vi "Tank_Monitoring.vi"(8 "Set state:":bool, 10 "Device":T1) -> (0 "Set":bool)   [LabVIEW 2011]
uses:
  Valve_Pump.ctl
  Tank Valves.ctl
  Ordered tank names.ctl
  Pumps_Valves_Dependencies_Global.vi
panel:
  out "Tank Names":string[](array[string])
  out "Happy Tank":bool[](array[boolean])
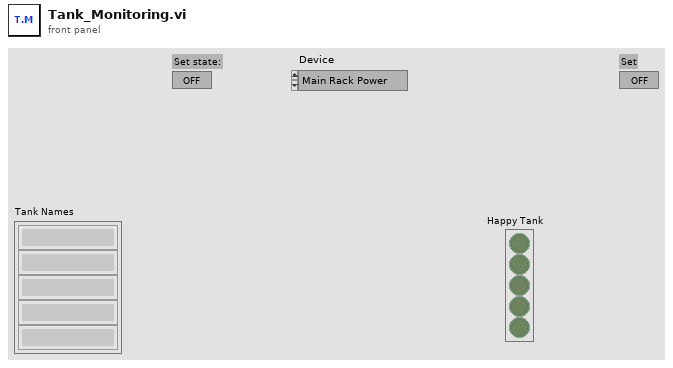
[diagram p1: front panel]
types:
  T1 = typedef "Valve_Pump.ctl" = enum16{"Main Rack Power", "Pump Power", "Valve Power", "V4", "V5", "V6", "V7", "V8", "V9", "V10", "V11", "V12", "V13", "V14", "V15", "V18", "V19", "V20", "V21", "V22", "V23", "V24", "V25", "V26", "V27", "V28", "V29", "V30", "V31", "V32", "V33", "V34", "Pump A", "Pump B", "Pump C", "Pump D"}
  T2 = typedef "Tank Valves.ctl" = enum16{"Salt Saturator", "Tank A", "Tank B", "Tank C", "Tank D"}
  T3 = typedef "Ordered tank names.ctl" = string[]
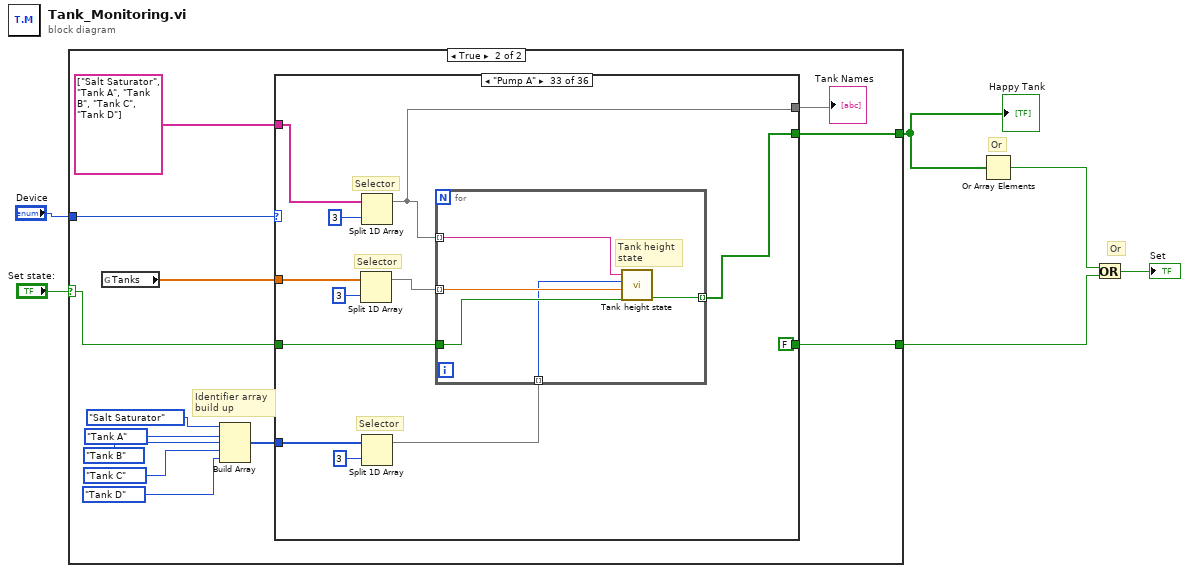
[diagram p0: block diagram]
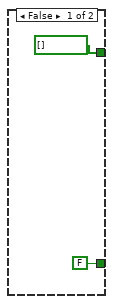
[diagram p2: hidden frame]
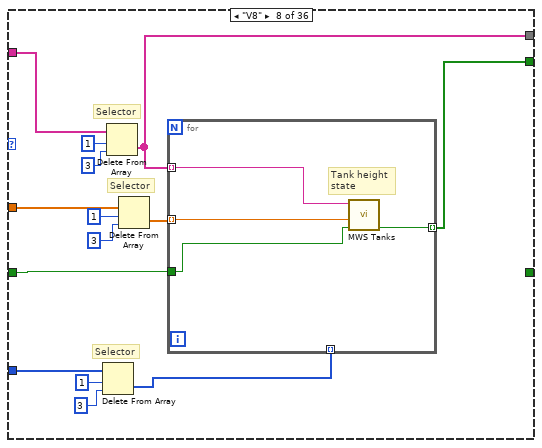
[diagram p10: hidden frame]
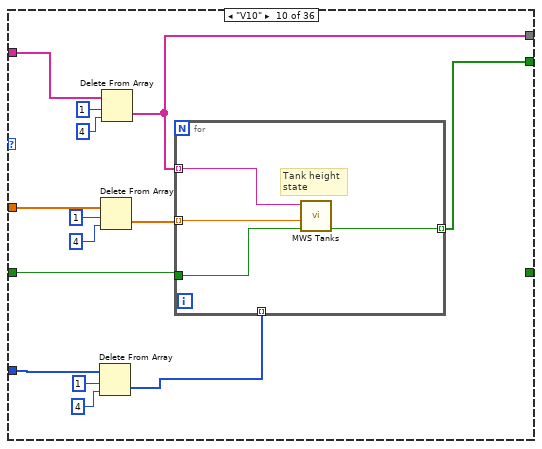
[diagram p12: hidden frame]
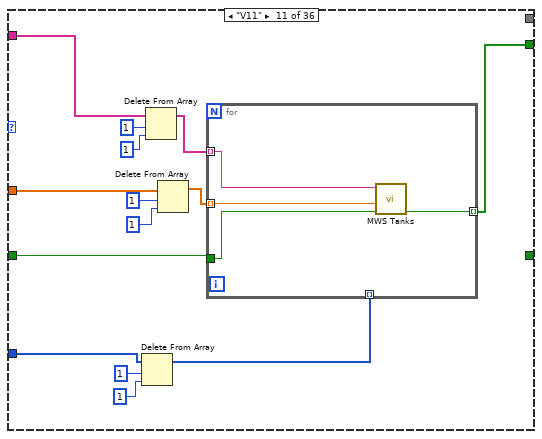
[diagram p13: hidden frame]
diagram:
  # "Or"
  # "Or"
  n1 = case shown="True" "Set state:" {
    selector: "Set state:" -> [_ w11]
    tunnel: [bool[] [] w20] -> w2
    tunnel: [FALSE w10] -> w5
    tunnel: "Device" -> [_ w9]
    frame False {
    }
    frame True {
      # "Identifier array\nbuild up"
      n2 = global read "Pumps_Valves_Dependencies_Global.vi" "Tanks"() -> (w21:dbl[])
      n3 = Build Array(Tank_Valves."Salt Saturator" ("Enum"), Tank_Valves."Tank A" ("Enum"), Tank_Valves."Tank B" ("Enum"), Tank_Valves."Tank C" ("Enum"), Tank_Valves."Tank D" ("Enum")) -> (w12:T2[])
      n4 = case shown="\"Pump A\"" w9 {
        tunnel: w21 -> [_ _ _ _ _ _ _ w35 _ w49 w68 _ _ _ _ _ _ _ _ _ _ _ _ _ _ _ _ _ _ _ _ _ w116 w131 w148 w160]
        tunnel: T3 ["Salt Saturator", "Tank A", "Tank B", "Tank C", "Tank D"] ("Ordered tank names") -> [_ _ _ _ _ _ _ w36 _ w52 w67 _ _ _ _ _ _ _ _ _ _ _ _ _ _ _ _ _ _ _ _ _ w112 w130 w147 w162]
        tunnel: [_ _ _ _ _ _ _ w33 _ w50 w66 _ _ _ _ _ _ _ _ _ _ _ _ _ _ _ _ _ _ _ _ _ w111 w129 w146 w170] -> w20
        tunnel: [_ _ _ _ _ _ _ w31 _ w51 _ _ _ _ _ _ _ _ _ _ _ _ _ _ _ _ _ _ _ _ _ _ w110 w124 w145 w161] -> w18
        tunnel: w12 -> [_ _ _ _ _ _ _ w32 _ w53 w70 _ _ _ _ _ _ _ _ _ _ _ _ _ _ _ _ _ _ _ _ _ w107 w127 w142 w166]
        tunnel: w11 -> [w22 w23 w24 w25 w26 w27 w28 w34 w47 w48 w69 w84 w85 w86 w87 w88 w89 w90 w91 w92 w93 w94 w95 w96 w97 w98 w99 w100 w101 w102 w103 w104 w109 w126 w140 w169]
        tunnel: [w22 w23 w24 w25 w26 w27 w28 _ w47 _ _ w84 w85 w86 w87 w88 w89 w90 w91 w92 w93 w94 w95 w96 w97 w98 w99 w100 w101 w102 w103 w104 FALSE FALSE FALSE FALSE] -> w10
        frame "Main Rack Power" {
        }
        frame "Pump Power" {
        }
        frame "Valve Power" {
        }
        frame "V4" {
        }
        frame "V5" {
        }
        frame "V6" {
        }
        frame "V7" {
        }
        frame "V8" {
          # "Selector"
          # "Selector"
          # "Selector"
          n5 = Delete From Array(array=w32, length=1, index=3) -> (deleted portion=w29:T2[])  [unwired: 1 out]
          n6 = Delete From Array(array=w36, length=1 ("index"), index=3 ("length")) -> (deleted portion=w31:T3)  [unwired: 1 out]
          n7 = Delete From Array(array=w35, length=1 ("index"), index=3 ("length")) -> (deleted portion=w30:dbl[])  [unwired: 1 out]
          n8 = for {
            tunnel: w30 -> [w45] mode=indexing
            tunnel: w31 -> [w44] mode=indexing
            tunnel: [w43] -> w33 mode=indexing
            tunnel: w29 -> [_] mode=indexing
            tunnel: w34 -> [w46]
            # "Tank height\nstate"
            n9 = call "MWS Tanks.vi"("Set state:"=w46, "Tank height"=w45, "Status Message"=w44) -> ("Set"=w43:bool)  [unwired: 8 in]
          }
        }
        frame "V9" {
        }
        frame "V10" {
          n10 = Delete From Array(array=w53, length=1, index=4) -> (deleted portion=w54:T2[])  [unwired: 1 out]
          n11 = Delete From Array(array=w49, length=1 ("index"), index=4 ("length")) -> (deleted portion=w55:dbl[])  [unwired: 1 out]
          n12 = Delete From Array(array=w52, length=1 ("index"), index=4 ("length")) -> (deleted portion=w51:T3)  [unwired: 1 out]
          n13 = for {
            tunnel: w55 -> [w64] mode=indexing
            tunnel: w51 -> [w63] mode=indexing
            tunnel: [w62] -> w50 mode=indexing
            tunnel: w54 -> [_] mode=indexing
            tunnel: w48 -> [w65]
            # "Tank height\nstate"
            n14 = call "MWS Tanks.vi"("Set state:"=w65, "Tank height"=w64, "Status Message"=w63) -> ("Set"=w62:bool)  [unwired: 8 in]
          }
        }
        frame "V11" {
          n15 = Delete From Array(array=w70, length=1, index=1) -> (array with subset deleted=w73:T2[])  [unwired: 1 out]
          n16 = Delete From Array(array=w67, length=1 ("index"), index=1 ("length")) -> (array with subset deleted=w76:T3)  [unwired: 1 out]
          n17 = Delete From Array(array=w68, length=1 ("index"), index=1 ("length")) -> (array with subset deleted=w79:dbl[])  [unwired: 1 out]
          n18 = for {
            tunnel: w79 -> [w82] mode=indexing
            tunnel: w76 -> [w80] mode=indexing
            tunnel: [w83] -> w66 mode=indexing
            tunnel: w73 -> [_] mode=indexing
            tunnel: w69 -> [w81]
            n19 = call "MWS Tanks.vi"("Set state:"=w81, "Tank height"=w82, "Status Message"=w80) -> ("Set"=w83:bool)  [unwired: 8 in]
          }
        }
        frame "V12" {
        }
        frame "V13" {
        }
        frame "V14" {
        }
        frame "V15" {
        }
        frame "V18" {
        }
        frame "V19" {
        }
        frame "V20" {
        }
        frame "V21" {
        }
        frame "V22" {
        }
        frame "V23" {
        }
        frame "V24" {
        }
        frame "V25" {
        }
        frame "V26" {
        }
        frame "V27" {
        }
        frame "V28" {
        }
        frame "V29" {
        }
        frame "V30" {
        }
        frame "V31" {
        }
        frame "V32" {
        }
        frame "V33" {
        }
        frame "V34" {
        }
        frame "Pump A" {
          # "Selector"
          # "Selector"
          # "Selector"
          n20 = Split 1D Array(array=w116, index=3) -> (first subarray=w115:dbl[])  [unwired: 1 out]
          n21 = Split 1D Array(array=w112, index=3) -> (first subarray=w110:T3)  [unwired: 1 out]
          n22 = Split 1D Array(array=w107, index=3) -> (first subarray=w106:T2[])  [unwired: 1 out]
          n23 = for {
            tunnel: w115 -> [w120] mode=indexing
            tunnel: w110 -> [w119] mode=indexing
            tunnel: w109 -> [w121]
            tunnel: [w118] -> w111 mode=indexing
            tunnel: w106 -> [w117] mode=indexing
            # "Tank height\nstate"
            n24 = call "Tank height state.vi"("Set state:"=w121, "Tank height"=w120, "Tank Valves"=w117, "Tank name"=w119) -> ("State"=w118:bool)  [unwired: 6 in]
          }
        }
        frame "Pump B" {
          # "Selector"
          # "Selector"
          # "Selector"
          n25 = Split 1D Array(array=w127, index=1) -> (second subarray=w122:T2[])  [unwired: 1 out]
          n26 = Split 1D Array(array=w131, index=1) -> (second subarray=w123:dbl[])  [unwired: 1 out]
          n27 = Split 1D Array(array=w130, index=1) -> (second subarray=w124:T3)  [unwired: 1 out]
          n28 = for {
            tunnel: w123 -> [w138] mode=indexing
            tunnel: w124 -> [w137] mode=indexing
            tunnel: [w136] -> w129 mode=indexing
            tunnel: w122 -> [w135] mode=indexing
            tunnel: w126 -> [w134]
            # "Tank height\nstate"
            n29 = call "Tank height state.vi"("Set state:"=w134, "Tank height"=w138, "Tank Valves"=w135, "Tank name"=w137) -> ("State"=w136:bool)  [unwired: 6 in]
          }
        }
        frame "Pump C" {
          # "Selector"
          # "Selector"
          # "Selector"
          n30 = Split 1D Array(array=w148, index=3) -> (second subarray=w144:dbl[])  [unwired: 1 out]
          n31 = Split 1D Array(array=w147, index=3) -> (second subarray=w145:T3)  [unwired: 1 out]
          n32 = Split 1D Array(array=w142, index=3) -> (second subarray=w141:T2[])  [unwired: 1 out]
          n33 = for {
            tunnel: w144 -> [w155] mode=indexing
            tunnel: w145 -> [w154] mode=indexing
            tunnel: [w153] -> w146 mode=indexing
            tunnel: w141 -> [w152] mode=indexing
            tunnel: w140 -> [w151]
            # "Tank height\nstate"
            n34 = call "Tank height state.vi"("Set state:"=w151, "Tank height"=w155, "Tank Valves"=w152, "Tank name"=w154) -> ("State"=w153:bool)  [unwired: 6 in]
          }
        }
        frame "Pump D" {
          # "Selector"
          # "Selector"
          # "Selector"
          n35 = Delete From Array(array=w166, length=1, index=1) -> (array with subset deleted=w165:T2[])  [unwired: 1 out]
          n36 = Delete From Array(array=w162, length=1 ("index"), index=1 ("length")) -> (array with subset deleted=w161:T3)  [unwired: 1 out]
          n37 = Delete From Array(array=w160, length=1 ("index"), index=1 ("length")) -> (array with subset deleted=w157:dbl[])  [unwired: 1 out]
          n38 = for {
            tunnel: w157 -> [w175] mode=indexing
            tunnel: w161 -> [w174] mode=indexing
            tunnel: [w173] -> w170 mode=indexing
            tunnel: w165 -> [w172] mode=indexing
            tunnel: w169 -> [w171]
            # "Tank height\nstate"
            n39 = call "Tank height state.vi"("Set state:"=w171, "Tank height"=w175, "Tank Valves"=w172, "Tank name"=w174) -> ("State"=w173:bool)  [unwired: 6 in]
          }
        }
      }
      "Tank Names" <- w18
    }
  }
  "Happy Tank" <- w2
  n40 = Or Array Elements(Boolean array=w2) -> (logical OR=w6:bool)
  n41 = Or(x=w6, y=w5) -> (x .or. y?=→"Set":bool)
